vi "create table.vi"(9 "columns type (real)":string="real", 10 "columns":string[](array[string]), 11 "table name":string="XQ") -> (3 "create table parameters":string)   [LabVIEW 2019, in "PostgreSQL.lvlib"]
uses:
  PostgreSQL.lvlib
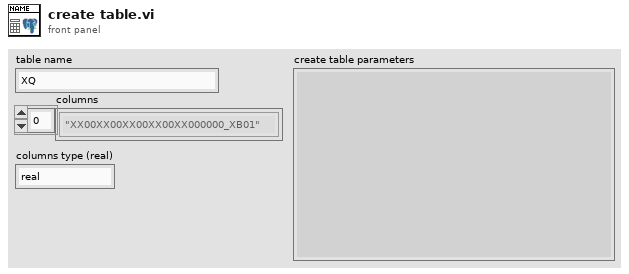
[diagram p1: front panel]
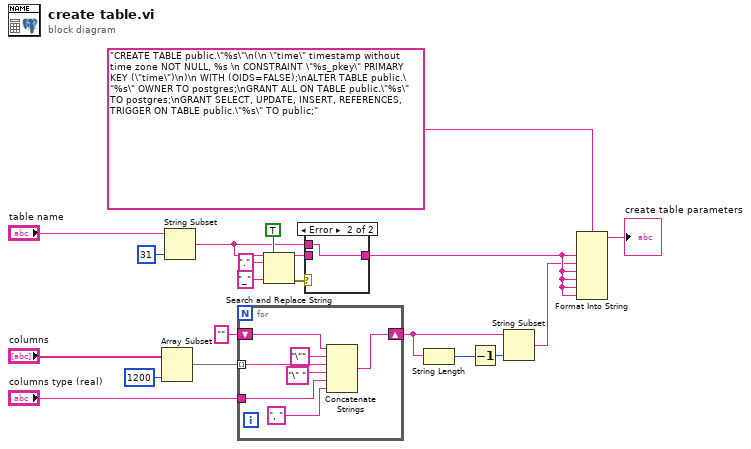
[diagram p0: block diagram]
diagram:
  n1 = Array Subset(array="columns", length=1200) -> (w8:string[])  [unwired: 1 in]
  n2 = String Subset(string="table name", length (rest)=31 ("offset (0)")) -> (substring=w14:string)  [unwired: 1 in]
  n3 = for {
    tunnel: w8 -> [w25] mode=indexing
    shift-right: [w23] -> w3
    shift-left: "" ("result string") -> [w24]
    tunnel: "columns type (real)" -> [w21]
    n4 = Concatenate Strings(w24, "\"" ("string"), w25, "\" " ("string"), w21, ", ") -> (w23:string)
  }
  n5 = Search and Replace String(replace all?=TRUE ("replace all? (F)"), input string=w14, search string=".", replace string="_" ("replace string (\"\")")) -> (result string=w17:string, error out=w18:errorcluster)  [unwired: 4 in, 2 out]
  n6 = case shown="Error" w18 {
    tunnel: w17 -> [w28 _]
    tunnel: [w28 w29] -> w7
    tunnel: w14 -> [_ w29]
    frame No Error {
    }
    frame Error {
    }
  }
  n7 = String Length(string=w3) -> (length=w2:i32)
  n8 = Decrement(x=w2) -> (x-1=w16:i32)
  n9 = String Subset(string=w3, length (rest)=w16) -> (substring=w6:string)  [unwired: 1 in]
  n10 = Format Into String(format string="CREATE TABLE public.\"%s\"\n(\n \"time\" timestamp without time zone NOT NULL, %s \n CONSTRAINT \"%s_pkey\" PRIMARY KEY (\"time\")\n)\n WITH (OIDS=FALSE);\nALTER TABLE public.\"%s\" OWNER TO postgres;\nGRANT ALL ON TABLE public.\"%s\" TO postgres;\nGRANT SELECT, UPDATE, INSERT, REFERENCES, TRIGGER ON TABLE public.\"%s\" TO public;", w7, w6, w7, w7, w7, w7) -> (resulting string=→"create table parameters":string)  [unwired: 2 in, 1 out]
